vi "Write Multi-Channel Records.vi"(7 "Group":string, 8 "error in (no error)":errorcluster, 9 "Data":dbl[][](array[numeric]), 10 "Channels":string[](array[string]), 11 "Report Generator in":refnum<class "Report Generator.lvclass">) -> (0 "error out":errorcluster, 3 "Report Generator out":refnum<class "Report Generator.lvclass">)   [LabVIEW 2023, in "Report Generator.lvlib" / "Report Generator.lvclass"]
doc: "Override this VI\nWrite Multiple Channel Data to report\n\n<b>Group</b> This is the instrument/device generating the data records\n<b>Channels</b> String name of channels contained in the Group & Data\n<b>Data</b> 2-d Array of Data to be logged in to the report."
uses:
  Library/Report Generator.lvclass
  Library/Report Generator.lvclass/Report Generator.ctl
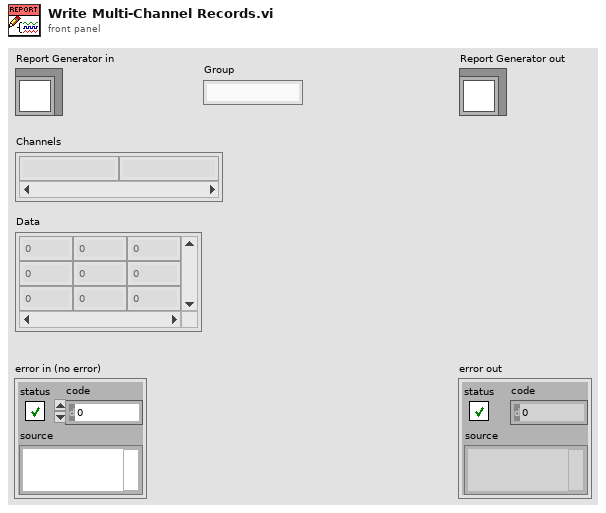
[diagram p1: front panel]
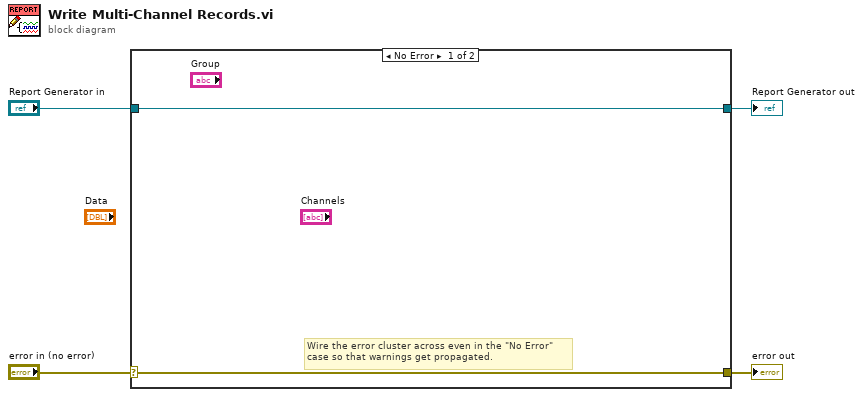
[diagram p0: block diagram]
diagram:
  n1 = case shown="No Error" "error in (no error)" {
    selector: "error in (no error)" -> [w5 w8]
    tunnel: [w5 w8] -> w3
    tunnel: [w6 w7] -> w1
    tunnel: "Report Generator in" -> [w6 w7]
    frame No Error {
      # "Wire the error cluster across even in the \"No Error\"\ncase so that warnings get propagated."
    }
    frame Error {
    }
  }
  "error out" <- w3
  "Report Generator out" <- w1
